vi "I.vi"(7 "Q":dbl, 8 "C_reg":dbl, 9 "C":dbl, 10 "L":dbl, 11 "f":dbl) -> (3 "I":dbl)   [LabVIEW 2020]
doc: "SubVI wyznacza natężenie prądu zwracane przez Q-metr."
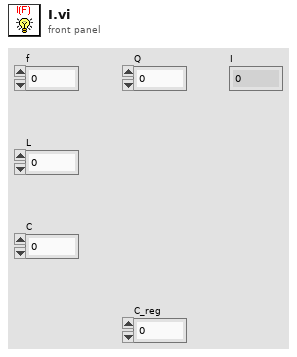
[diagram p1: front panel]
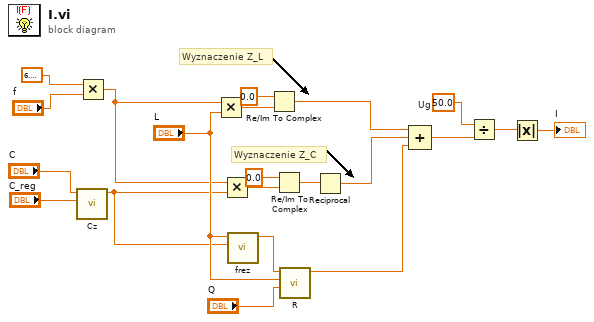
[diagram p0: block diagram]
diagram:
  w11 = 50.0  # Ug
  # "Wyznaczenie Z_C"
  # "Wyznaczenie Z_L"
  n1 = call "Cz.vi"("C_reg"="C_reg", "C"="C") -> ("Cz"=w12:dbl)  [unwired: 9 in]
  n2 = Multiply(x=6.283185307179586, y="f") -> (x*y=w7:dbl)
  n3 = Multiply(x=w7, y="L") -> (x*y=w3:dbl)
  n4 = Multiply(x=w7, y=w12) -> (x*y=w8:dbl)
  n5 = call "frez.vi"("Cz"=w12, "L"="L") -> ("f_rez"=w20:dbl)  [unwired: 9 in]
  n6 = Re/Im To Complex(1:w3, 2:0.0 ("x")) -> (0:w16:cdb)
  n7 = Re/Im To Complex(1:w8, 2:0.0 ("x")) -> (0:w10:cdb)
  n8 = call "R.vi"("Q"="Q", "L"="L", "f_rez"=w20) -> ("R"=w18:cdb)  [unwired: 8 in]
  n9 = Reciprocal(x=w10) -> (1/x=w17:cdb)
  n10 = Compound Arithmetic op=ADD(w16, w17, w18) -> (w15:cdb)
  n11 = Divide(x=w11, y=w15) -> (x/y=w1:cdb)
  n12 = Absolute Value(x=w1) -> (abs(x)=→"I":dbl)
